vi "DAQ Assist_AD.vi"() -> ()   [LabVIEW 2010]
panel:
  in  "rate":dbl=256.0
  in  "stop":bool
  out "ms":u32
  out "Waveform Chart":dbl[](graph)
  in  "stop (F)":bool
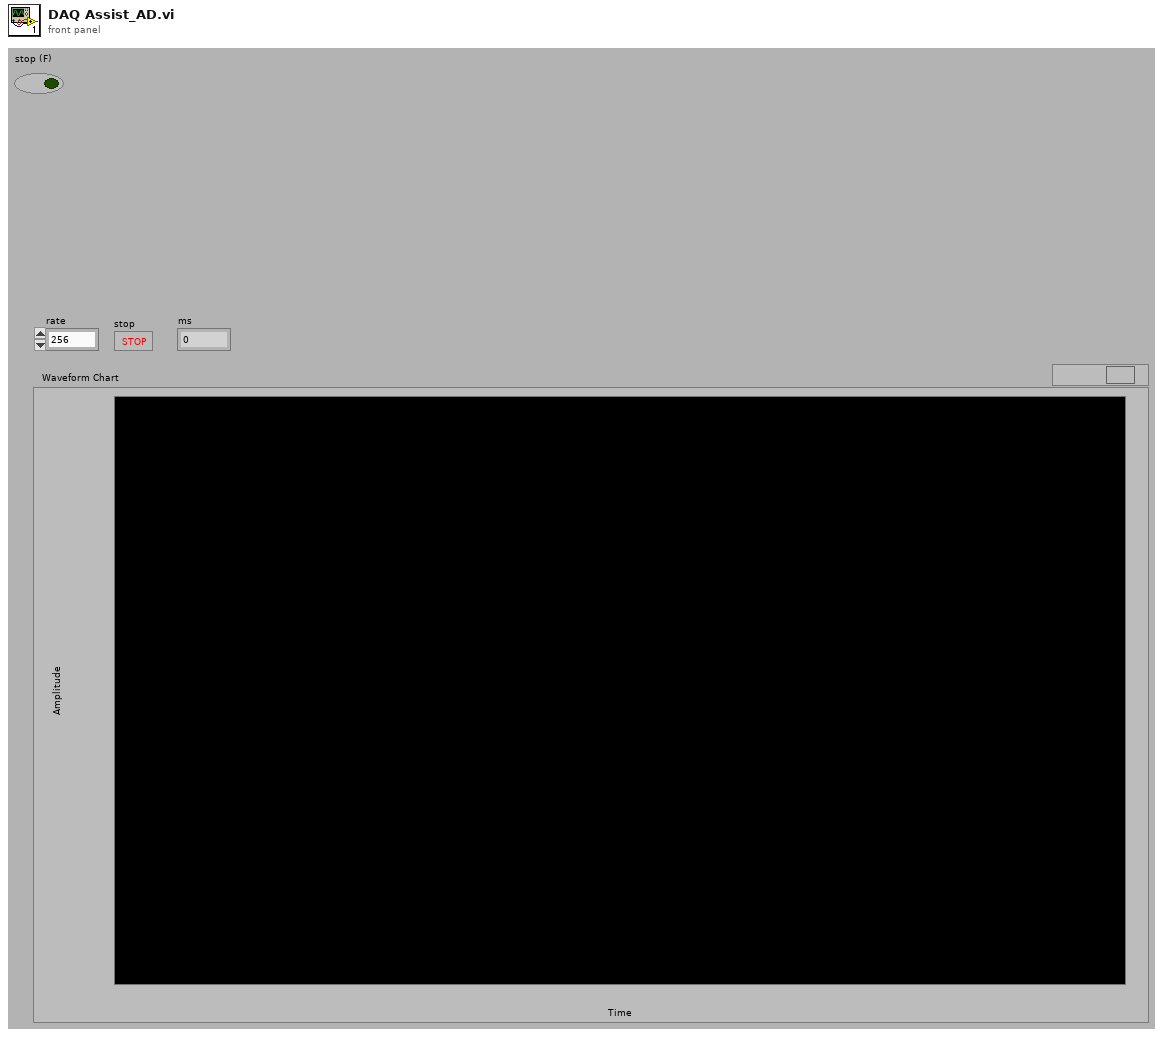
[diagram p1: front panel]
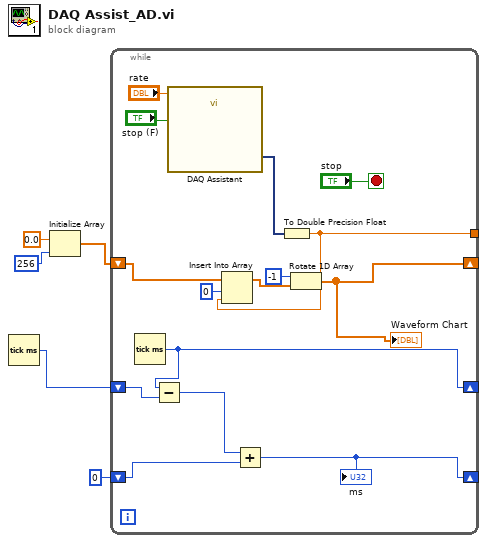
[diagram p0: block diagram]
diagram:
  n1 = Tick Count (ms)() -> (millisecond timer value=w2:u32)
  n2 = Initialize Array(0.0 ("element"), 256 ("dimension size")) -> (w3:dbl[])
  n3 = while {
    tunnel: [w16] -> _
    shift-right: [w13] -> _
    shift-left: w3 -> [w18]
    shift-right: [w8] -> _
    shift-left: u32 0 -> [w11]
    shift-right: [w10] -> _
    shift-left: w2 -> [w9]
    stop <- "stop" stop-if-true
    n4 = Tick Count (ms)() -> (millisecond timer value=w10:u32)
    n5 = Subtract(x=w10, y=w9) -> (x-y=w12:u32)
    n6 = call "DAQ Assistant"("rate"="rate", "stop (F)"="stop (F)") -> ("data"=w19:dynamicdata)  [unwired: 14 in, 3 out]
    n7 = Add(x=w12, y=w11) -> (x+y=w8:u32)
    "ms" <- w8
    n8 = To Double Precision Float(number=w19) -> (double precision float=w16:dbl)
    n9 = Insert Into Array(array=w18, index=0, new element=w16) -> (w15:dbl[])
    n10 = Rotate 1D Array(1:w15, 2:-1 ("n")) -> (0:w13:dbl[])
    "Waveform Chart" <- w13
  }
